vi "timer.vi"() -> ()   [LabVIEW 2015]
panel:
  in  "Stop":bool
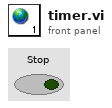
[diagram p1: front panel]
diagram:
